vi "gCode_analyseReceivedMessage.vi"(10 "UI_Data":T2={"controlTabState"=[], "pathToSTLFiles"=path "", "availableObjs"=[], "objectNames"=[], "addedObjs"=[], "selectedObj"={"Name"="", "objectFiles"=[], "center"={"X"=0.0, "Y"=0.0, "Z"=0.0}, "extent"={"X"=0.0, "Y"=0.0, "Z"=0.0}, "allowedMotion"=enum."XY", "mountOn"=enum."yArm", "Movements"=[], "extraInfo"=[], "hasPOI?"=FALSE, "POI"={"X"=0.0, "Y"=0.0, "Z"=0.0}, "posOffset"={"X"=0.0, "Y"=0.0, "Z"=0.0}, "referenceNum"=refnum}, "3DPictureObjRef"=refnum, "yPOI_0"={"X"=0.0, "Y"=0.0, "Z"=0.0}, "yPOI"={"X"=0.0, "Y"=0.0, "Z"=0.0}, "yPOI_Added?"=FALSE, "breadBoard_00"={"X"=0.0, "Y"=0.0, "Z"=0.0}, "breadBoardOriginOffset"={"X"=0.0, "Y"=0.0, "Z"=0.0}, "XYtranslateObjControls"=[], "ZtranslateObjControls"=[], "pBot_controls"=[], "pBot_VISA"="", "commandLog"="", "pBotConnected?"=FALSE, "pBot_currentEEPROMsettings"="", "realTimeInfoControls"=[], "pBot_tempSensor1"=0.0, "pBot_tempSensor2"=0.0, "realTimeInfoTextColor"=[], "disconnectPBot_Event"=refnum, "needToHomeY?"=FALSE, "pBot_relativePositioning"=FALSE, "pBot_minPos"={"X"=0.0, "Y"=0.0, "Z"=0.0}, "pBot_maxPos"={"X"=0.0, "Y"=0.0, "Z"=0.0}, "pBot_homeOffset"={"X"=0.0, "Y"=0.0, "Z"=0.0}, "textColorGreen"=9174826, "textColorRed"=16750216, "textColorGray"=9868950, "transVisualizationControls"=[], "needToHomeXY?"=FALSE, "pBot_minScanRegion"={"X"=0.0, "Y"=0.0, "Z"=0.0}, "pBot_maxScanRegion"={"X"=0.0, "Y"=0.0, "Z"=0.0}, "pBot_scanN"={"X"=0, "Y"=0, "Z"=0}, "connectedInstruments"=[], "isScanning?"=FALSE, "Wavelengths"=[], "usb2000p_controlRefs"=[], "3DPictureRef"=refnum}, 11 "pBotMessageData":T1={"commandID"=" ", "gCode"=" ", "extraInfo"=" ", "originatingCommandID"=" ", "error"={"status"=FALSE, "code"=0, "source"=""}}) -> (0 "error Out":errorcluster, 2 "UI_Data Out":T2={"controlTabState"=[], "pathToSTLFiles"=path "", "availableObjs"=[], "objectNames"=[], "addedObjs"=[], "selectedObj"={"Name"="", "objectFiles"=[], "center"={"X"=0.0, "Y"=0.0, "Z"=0.0}, "extent"={"X"=0.0, "Y"=0.0, "Z"=0.0}, "allowedMotion"=enum."XY", "mountOn"=enum."yArm", "Movements"=[], "extraInfo"=[], "hasPOI?"=FALSE, "POI"={"X"=0.0, "Y"=0.0, "Z"=0.0}, "posOffset"={"X"=0.0, "Y"=0.0, "Z"=0.0}, "referenceNum"=refnum}, "3DPictureObjRef"=refnum, "yPOI_0"={"X"=0.0, "Y"=0.0, "Z"=0.0}, "yPOI"={"X"=0.0, "Y"=0.0, "Z"=0.0}, "yPOI_Added?"=FALSE, "breadBoard_00"={"X"=0.0, "Y"=0.0, "Z"=0.0}, "breadBoardOriginOffset"={"X"=25.4, "Y"=12.7, "Z"=12.7}, "XYtranslateObjControls"=[], "ZtranslateObjControls"=[], "pBot_controls"=[], "pBot_VISA"="", "commandLog"="", "pBotConnected?"=FALSE, "pBot_currentEEPROMsettings"="", "realTimeInfoControls"=[], "pBot_tempSensor1"=0.0, "pBot_tempSensor2"=0.0, "realTimeInfoTextColor"=[], "disconnectPBot_Event"=refnum, "needToHomeY?"=FALSE, "pBot_relativePositioning"=FALSE, "pBot_minPos"={"X"=0.0, "Y"=0.0, "Z"=0.0}, "pBot_maxPos"={"X"=0.0, "Y"=0.0, "Z"=0.0}, "pBot_homeOffset"={"X"=0.0, "Y"=0.0, "Z"=0.0}, "textColorGreen"=9174826, "textColorRed"=16750216, "textColorGray"=9868950, "transVisualizationControls"=[], "needToHomeXY?"=FALSE, "pBot_minScanRegion"={"X"=0.0, "Y"=0.0, "Z"=0.0}, "pBot_maxScanRegion"={"X"=0.0, "Y"=0.0, "Z"=0.0}, "pBot_scanN"={"X"=0, "Y"=0, "Z"=0}, "connectedInstruments"=[], "isScanning?"=FALSE, "Wavelengths"=[], "usb2000p_controlRefs"=[], "3DPictureRef"=refnum}, 3 "messageOut":string)   [LabVIEW 2015]
uses:
  controls/UI Data.ctl
  processedObjectInfo.ctl
  controls/scanInstrumentInfo.ctl
  controls/pBotMessageData.ctl
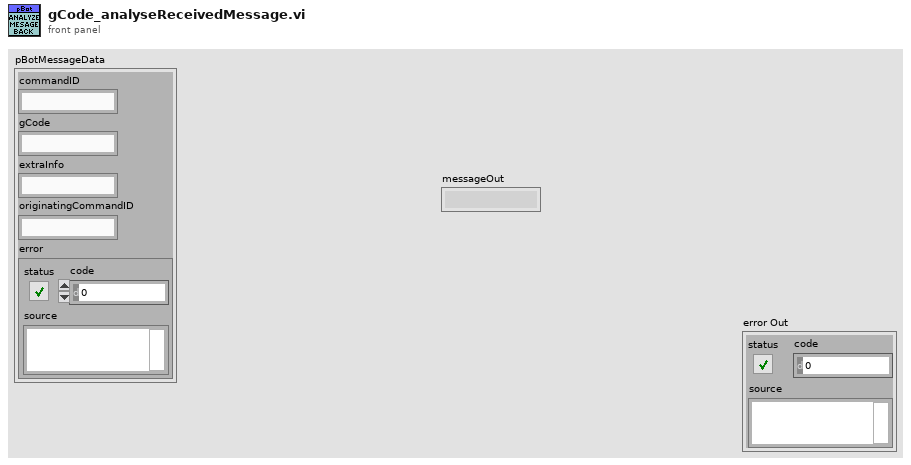
[diagram p1: front panel]
types:
  T1 = typedef "pBotMessageData.ctl" = cluster{"commandID":string, "gCode":string, "extraInfo":string, "originatingCommandID":string, "error":errorcluster}
  T2 = typedef "UI Data.ctl" = cluster{"controlTabState":bool[], "pathToSTLFiles":path, "availableObjs":T3[], "objectNames":string[], "addedObjs":T3[], "selectedObj":T3, "3DPictureObjRef":refnum<vi>, "yPOI_0":cluster{"X":dbl, "Y":dbl, "Z":dbl}, "yPOI":cluster{"X":dbl, "Y":dbl, "Z":dbl}, "yPOI_Added?":bool, "breadBoard_00":cluster{"X":dbl, "Y":dbl, "Z":dbl}, "breadBoardOriginOffset":cluster{"X":dbl, "Y":dbl, "Z":dbl}, "XYtranslateObjControls":refnum<vi>[], "ZtranslateObjControls":refnum<vi>[], "pBot_controls":refnum<vi>[], "pBot_VISA":refnum<visa-resource-name>, "commandLog":string, "pBotConnected?":bool, "pBot_currentEEPROMsettings":string, "realTimeInfoControls":refnum<vi>[], "pBot_tempSensor1":dbl, "pBot_tempSensor2":dbl, "realTimeInfoTextColor":u32[], "disconnectPBot_Event":refnum<user-event>, "needToHomeY?":bool, "pBot_relativePositioning":bool, "pBot_minPos":cluster{"X":dbl, "Y":dbl, "Z":dbl}, "pBot_maxPos":cluster{"X":dbl, "Y":dbl, "Z":dbl}, "pBot_homeOffset":cluster{"X":dbl, "Y":dbl, "Z":dbl}, "textColorGreen":u32, "textColorRed":u32, "textColorGray":u32, "transVisualizationControls":refnum<vi>[], "needToHomeXY?":bool, "pBot_minScanRegion":cluster{"X":sgl, "Y":sgl, "Z":sgl}, "pBot_maxScanRegion":cluster{"X":sgl, "Y":sgl, "Z":sgl}, "pBot_scanN":cluster{"X":u16, "Y":u16, "Z":u16}, "connectedInstruments":T4[], "isScanning?":bool, "Wavelengths":dbl[], "usb2000p_controlRefs":refnum<vi>[], "3DPictureRef":refnum<vi>}
  T3 = typedef "processedObjectInfo.ctl" = cluster{"Name":string, "objectFiles":cluster{"Location":path, "Color":cluster{"R":dbl, "G":dbl, "B":dbl, "A":dbl}}[], "center":cluster{"X":dbl, "Y":dbl, "Z":dbl}, "extent":cluster{"X":dbl, "Y":dbl, "Z":dbl}, "allowedMotion":enum16{"XY", "Z"}, "mountOn":enum16{"yArm", "breadBoard"}, "Movements":cluster{"Type":enum16{"rr", "ra", "tr", "ta"}, "vector":cluster{"X":dbl, "Y":dbl, "Z":dbl}, "scalar":dbl}[], "extraInfo":cluster{"parameter":string, "dataType":string, "vector":cluster{"X":dbl, "Y":dbl, "Z":dbl}, "scalar":dbl}[], "hasPOI?":bool, "POI":cluster{"X":dbl, "Y":dbl, "Z":dbl}, "posOffset":cluster{"X":dbl, "Y":dbl, "Z":dbl}, "referenceNum":refnum<vi>}
  T4 = typedef "scanInstrumentInfo.ctl" = cluster{"Name":string, "VISAname":refnum<visa-resource-name>, "1D_dataArraySize":u16, "extraInfo":variant, "error":errorcluster}
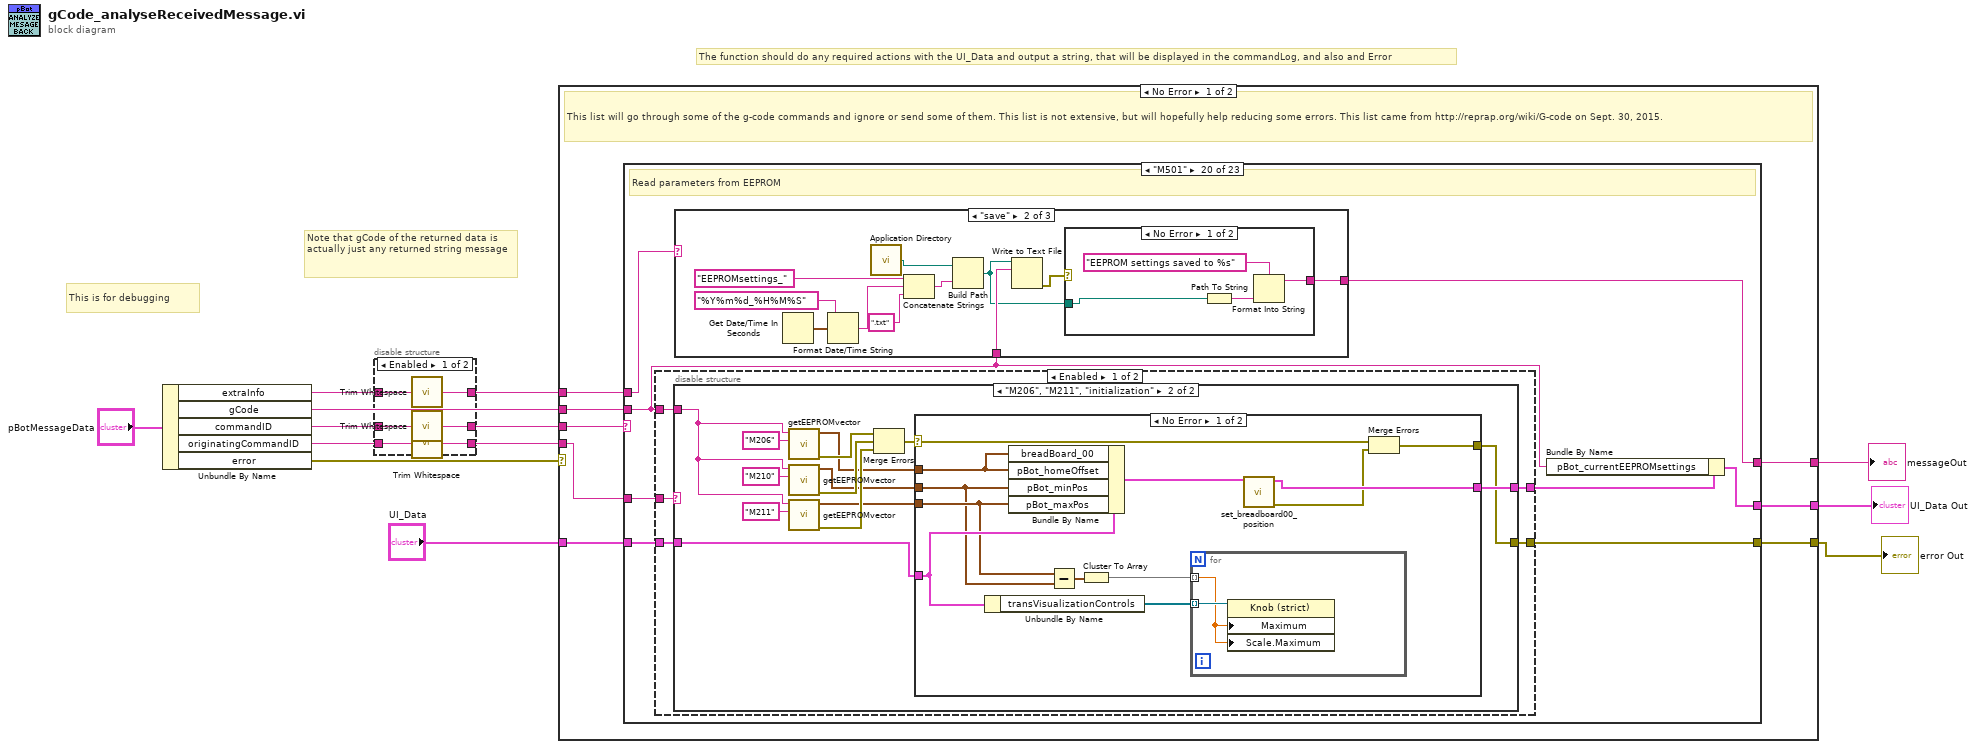
[diagram p0: block diagram]
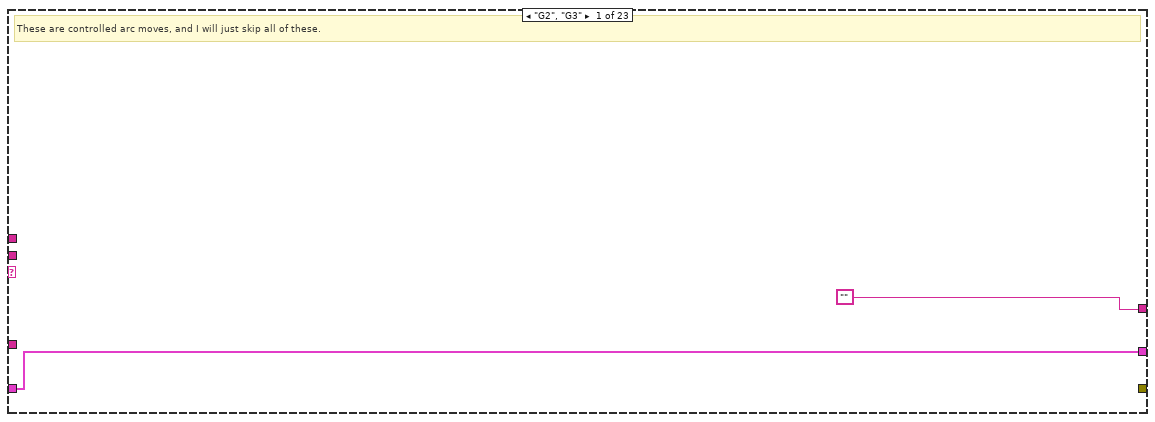
[diagram p3: hidden frame]
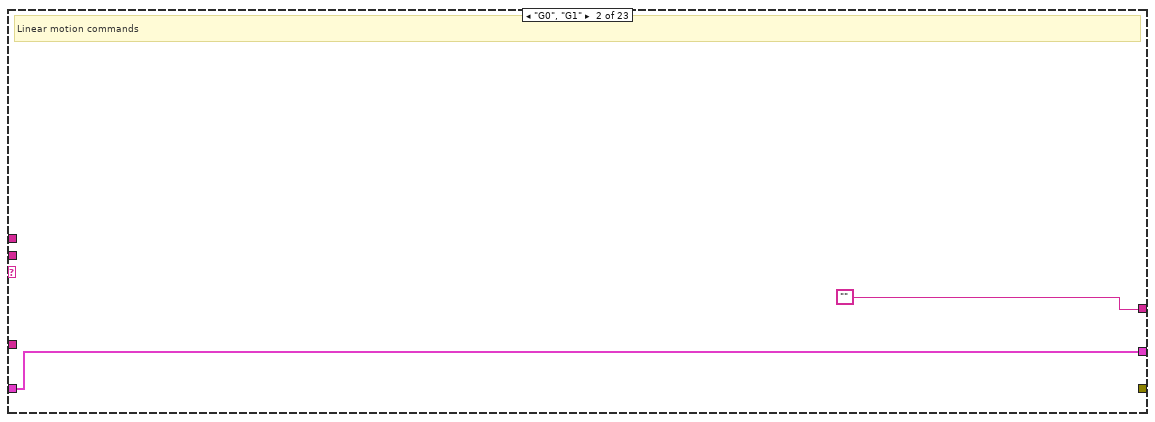
[diagram p4: hidden frame]
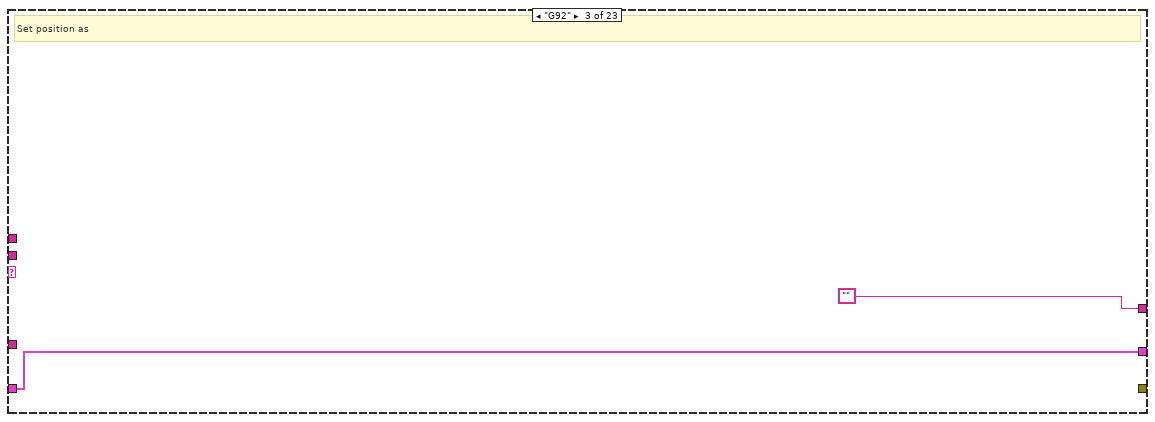
[diagram p5: hidden frame]
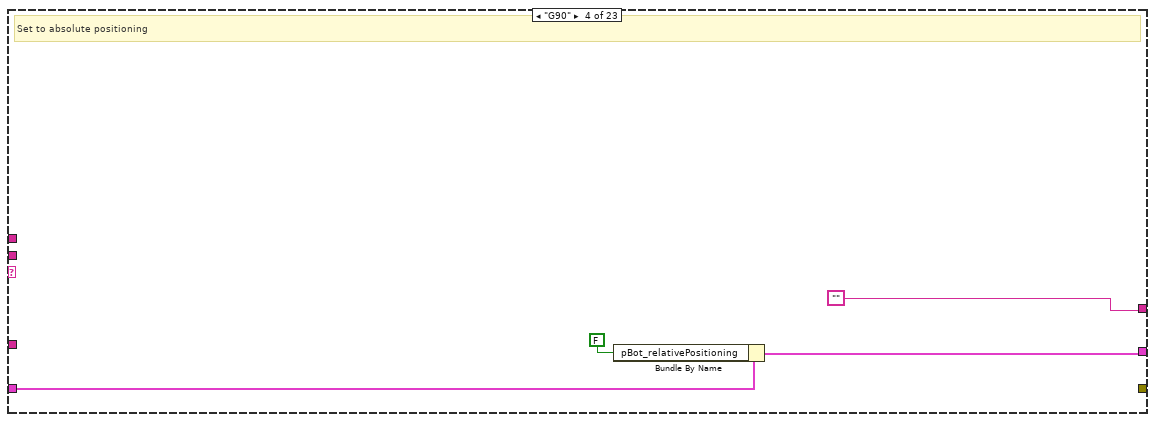
[diagram p6: hidden frame]
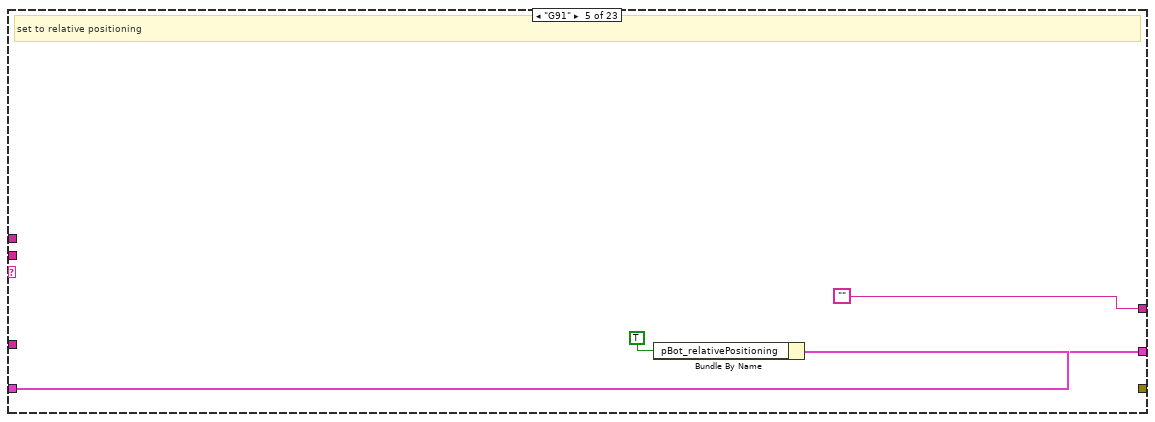
[diagram p7: hidden frame]
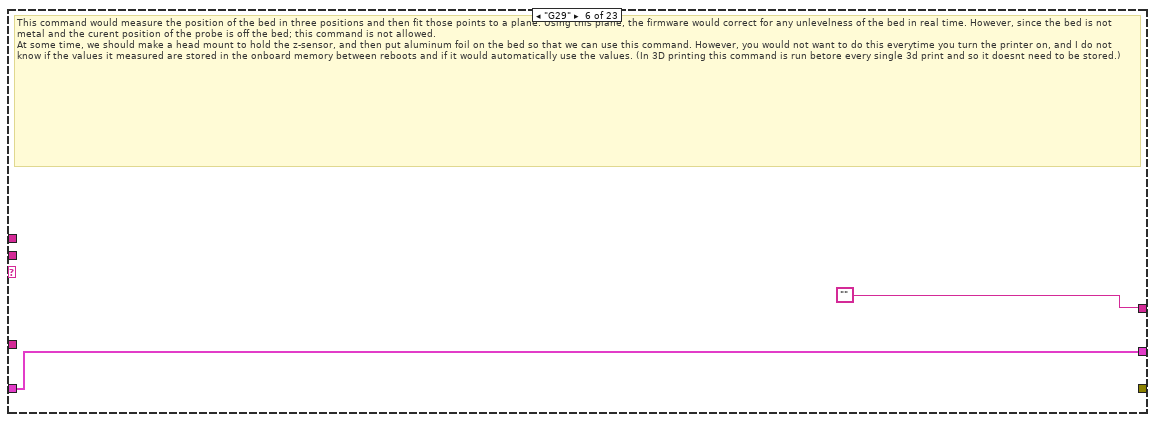
[diagram p8: hidden frame]
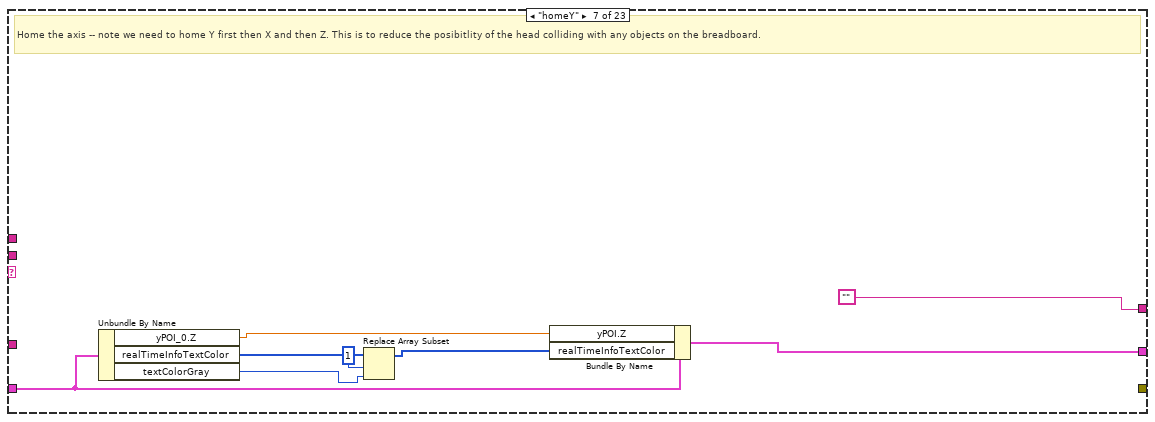
[diagram p9: hidden frame]
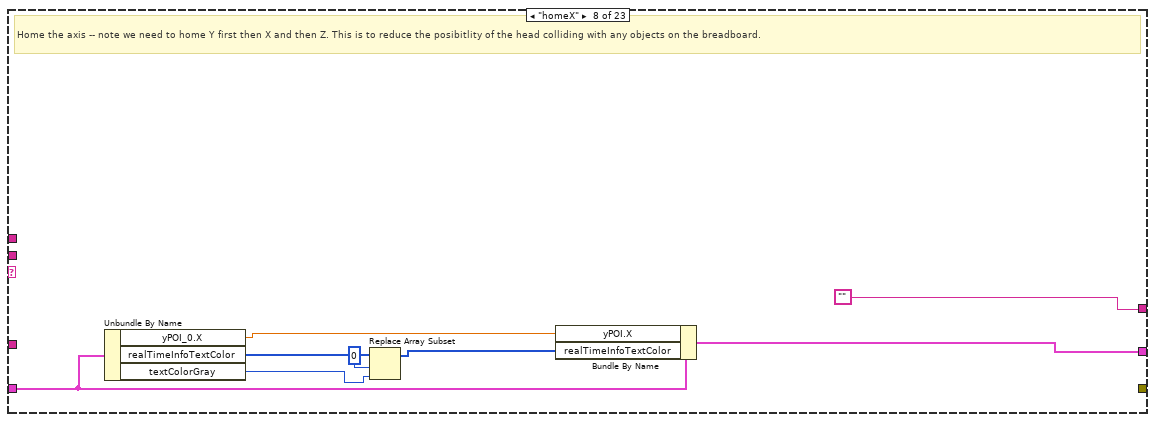
[diagram p10: hidden frame]
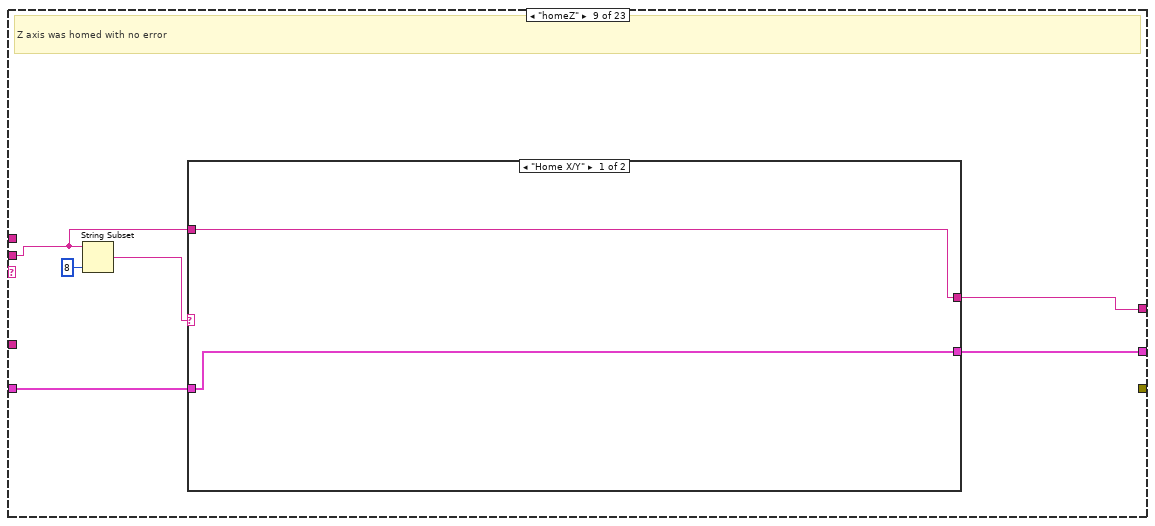
[diagram p11: hidden frame]
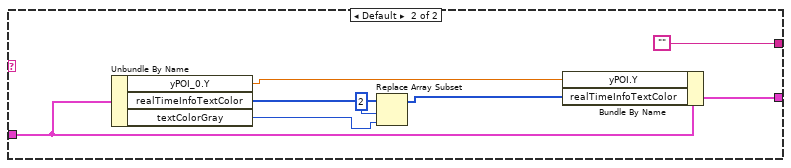
[diagram p12: hidden frame]
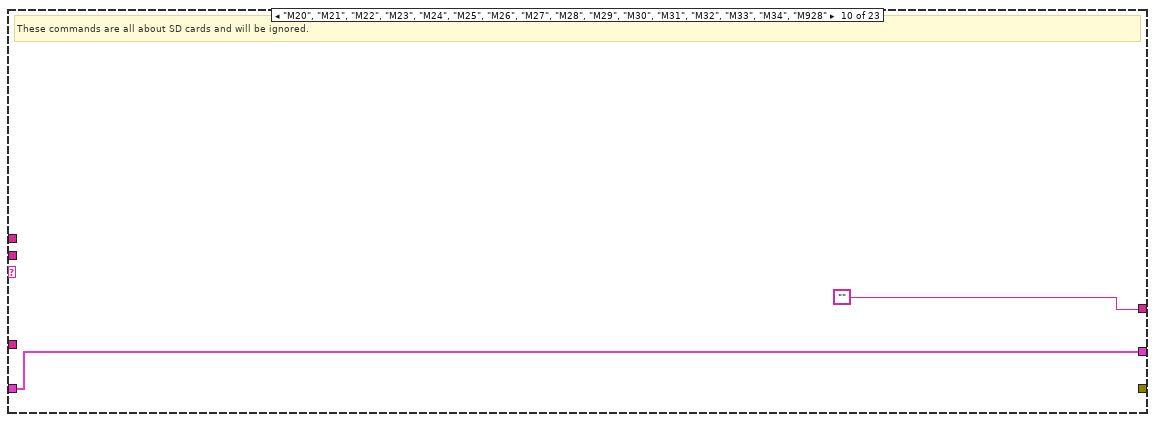
[diagram p13: hidden frame]
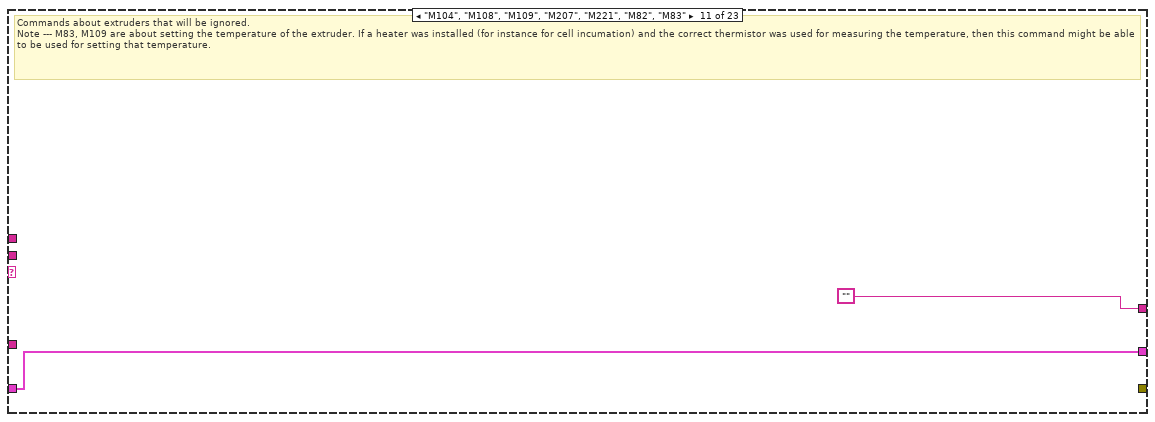
[diagram p14: hidden frame]
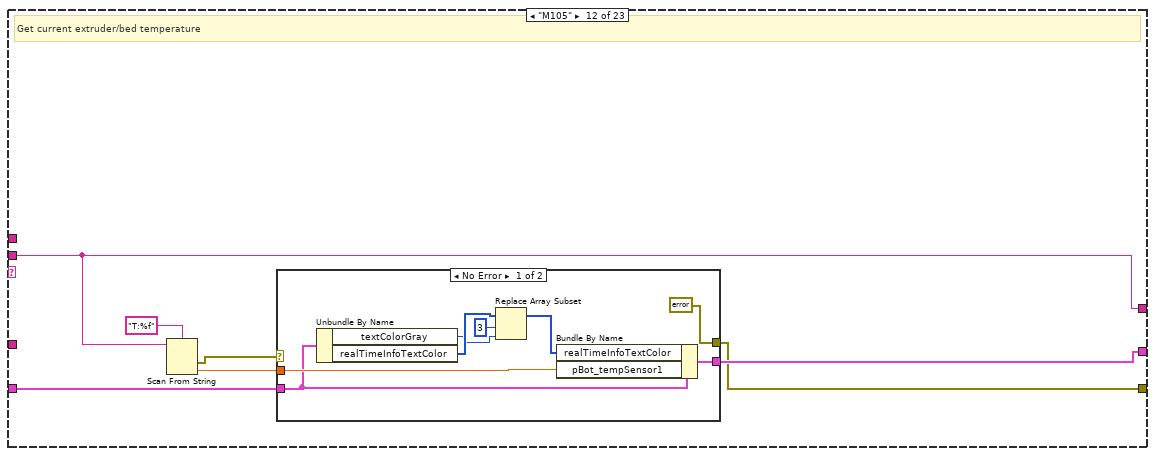
[diagram p15: hidden frame]
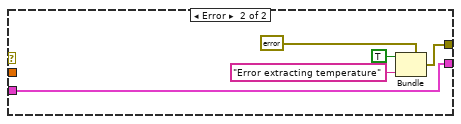
[diagram p16: hidden frame]
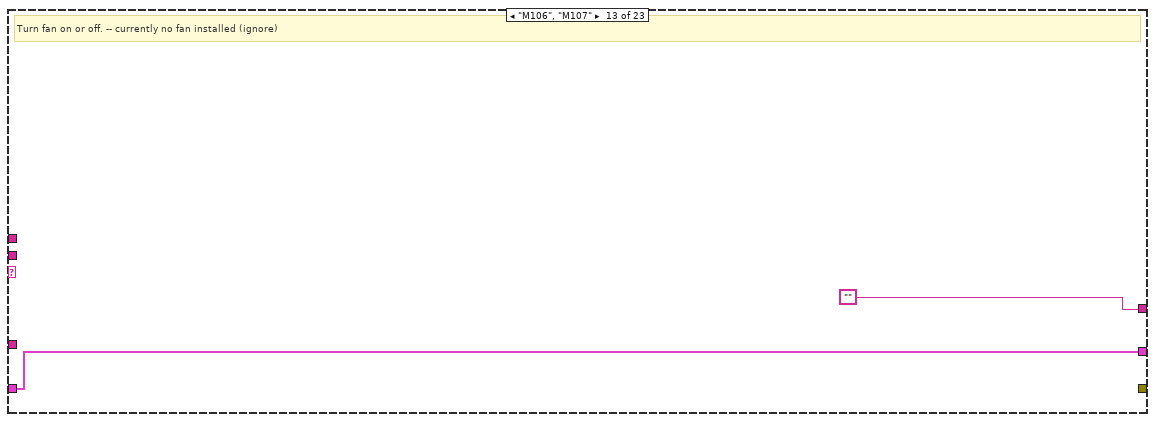
[diagram p17: hidden frame]
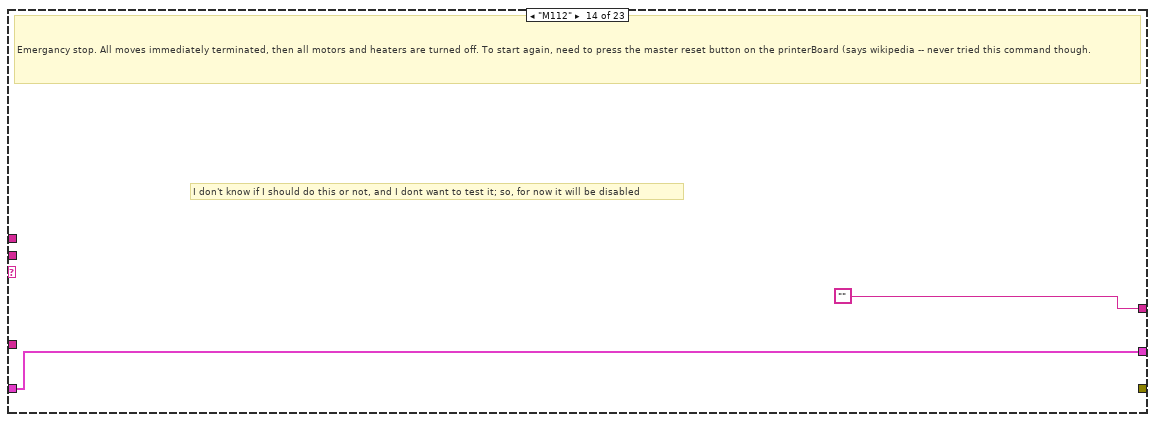
[diagram p18: hidden frame]
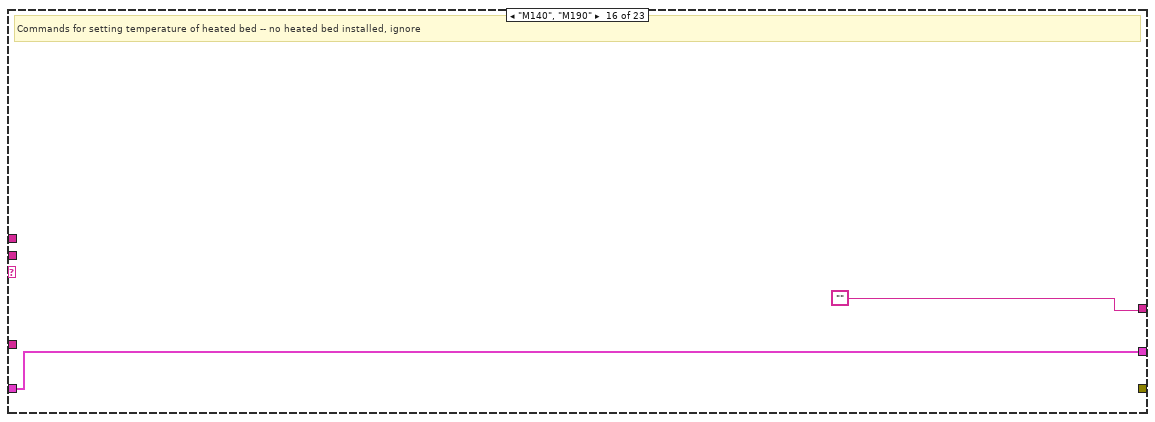
[diagram p20: hidden frame]
diagram:
  # "This is for debugging"
  # "Note that gCode of the returned data is actually just any returned string message"
  # "The function should do any required actions with the UI_Data and output a string, that will be displayed in the commandLog, and also and Error"
  n1 = Unbundle By Name("pBotMessageData") -> ("extraInfo"=w2:string, "gCode"=w11:string, "commandID"=w3:string, "originatingCommandID"=w6:string, "error"=w13:errorcluster)
  n2 = disable-structure shown="Enabled" {
    disable-tunnel: w6 -> [w19 w20]
    disable-tunnel: [w18 w20] -> w5
    disable-tunnel: [w17 w21] -> w4
    disable-tunnel: w3 -> [w16 w21]
    disable-tunnel: w2 -> [w15 w22]
    disable-tunnel: [w14 w22] -> w1
    frame Enabled {
      n3 = call <vilib>:"Trim Whitespace.vi"("string"=w15) -> ("trimmed string"=w14:string)  [unwired: 1 in]
      n4 = call <vilib>:"Trim Whitespace.vi"("string"=w16) -> ("trimmed string"=w17:string)  [unwired: 1 in]
      n5 = call <vilib>:"Trim Whitespace.vi"("string"=w19) -> ("trimmed string"=w18:string)  [unwired: 1 in]
    }
    frame Disabled {
    }
  }
  n6 = case shown="No Error" w13 {
    selector: w13 -> [_ w188]
    tunnel: [w28 w191] -> w10
    tunnel: w4 -> [w30 w193]
    tunnel: "UI_Data" -> [w29 w192]
    tunnel: w11 -> [w27 w190]
    tunnel: [w26 w189] -> w8
    tunnel: [w25 w187] -> w9
    tunnel: w1 -> [w24 _]
    tunnel: w5 -> [w23 _]
    frame No Error {
      # "This list will go through some of the g-code commands and ignore or send some of them. This list is not extensive, but will hopefully help reducing some errors. This list came from http://reprap.org/wiki/G-code on Sept. 30, 2015."
      n7 = case shown="\"M501\"" w30 {
        tunnel: w29 -> [w32 w34 w36 w40 w43 w46 w50 w57 w68 w80 w81 w87 w104 w106 w107 w110 w111 w114 w115 w124 w182 w184 w186]
        tunnel: [w32 w34 w36 w39 w42 w46 w49 w58 w67 w80 w81 w85 w104 w106 w107 w110 w111 w114 w115 w122 w182 w184 w186] -> w25
        tunnel: ["" "" "" "" "" "" "" "" w66 "" "" w83 "" "" w108 "" "" "" w116 w121 w181 "" w185] -> w28
        tunnel: w27 -> [_ _ _ _ _ _ _ _ w63 _ _ w83 _ _ w108 _ _ _ w116 w119 w181 _ w185]
        tunnel: [_ _ _ _ _ _ _ _ _ _ _ w84 _ _ _ _ _ _ _ w120 _ _ _] -> w26
        tunnel: w24 -> [_ _ _ _ _ _ _ _ _ _ _ _ _ _ _ _ _ _ _ w118 _ _ _]
        tunnel: w23 -> [_ _ _ _ _ _ _ _ _ _ _ _ _ _ _ _ _ _ _ w117 _ _ _]
        frame "G2", "G3" {
          # "These are controlled arc moves, and I will just skip all of these."
        }
        frame "G0", "G1" {
          # "Linear motion commands"
        }
        frame "G92" {
          # "Set position as"
        }
        frame "G90" {
          # "Set to absolute positioning"
          n8 = Bundle By Name(cluster=w40, "pBot_relativePositioning"=FALSE) -> (w39:T2)
        }
        frame "G91" {
          # "set to relative positioning"
          n9 = Bundle By Name(cluster=w43, "pBot_relativePositioning"=TRUE) -> (w42:T2)
        }
        frame "G29" {
          # "This command would measure the position of the bed in three positions and then fit those points to a plane. Using this plane, the firmware would correct for any unlevelness of the bed in real time. However, since the bed is not metal and the curent position of the probe is off the bed; this command is not allowed.\nAt some time, we should make a head mount to hold the z-sensor, and then put aluminum foil on the bed so that we can use this command. However, you would not want to do this everytime you turn the printer on, and I do not know if the values it measured are stored in the onboard memory between reboots and if it would automatically use the values. (In 3D printing this command is run betore every single 3d print and so it doesnt need to be stored.)"
        }
        frame "homeY" {
          # "Home the axis -- note we need to home Y first then X and then Z. This is to reduce the posibitlity of the head colliding with any objects on the breadboard."
          n10 = Unbundle By Name(w50) -> ("yPOI_0.Z"=w47:dbl, "realTimeInfoTextColor"=w54:u32[], "textColorGray"=w52:u32)
          n11 = Replace Array Subset(array=w54, new element=w52, index=1) -> (w51:u32[])
          n12 = Bundle By Name(cluster=w50, "yPOI.Z"=w47, "realTimeInfoTextColor"=w51) -> (w49:T2)
        }
        frame "homeX" {
          # "Home the axis -- note we need to home Y first then X and then Z. This is to reduce the posibitlity of the head colliding with any objects on the breadboard."
          n13 = Unbundle By Name(w57) -> ("yPOI_0.X"=w55:dbl, "realTimeInfoTextColor"=w62:u32[], "textColorGray"=w60:u32)
          n14 = Replace Array Subset(array=w62, new element=w60, index=0) -> (w59:u32[])
          n15 = Bundle By Name(cluster=w57, "yPOI.X"=w55, "realTimeInfoTextColor"=w59) -> (w58:T2)
        }
        frame "homeZ" {
          # "Z axis was homed with no error"
          n16 = String Subset(string=w63, length (rest)=8 ("length (rest)")) -> (substring=w64:string)  [unwired: 1 in]
          n17 = case shown="\"Home X/Y\"" w64 {
            tunnel: w68 -> [w70 w78]
            tunnel: [w70 w73] -> w67
            tunnel: [w69 ""] -> w66
            tunnel: w63 -> [w69 _]
            frame "Home X/Y" {
            }
            frame Default {
              n18 = Unbundle By Name(w78) -> ("yPOI_0.Y"=w71:dbl, "realTimeInfoTextColor"=w77:u32[], "textColorGray"=w75:u32)
              n19 = Replace Array Subset(array=w77, new element=w75, index=2) -> (w74:u32[])
              n20 = Bundle By Name(cluster=w78, "yPOI.Y"=w71, "realTimeInfoTextColor"=w74) -> (w73:T2)
            }
          }
        }
        frame "M20", "M21", "M22", "M23", "M24", "M25", "M26", "M27", "M28", "M29", "M30", "M31", "M32", "M33", "M34", "M928" {
          # "These commands are all about SD cards and will be ignored."
        }
        frame "M104", "M108", "M109", "M207", "M221", "M82", "M83" {
          # "Commands about extruders that will be ignored.\nNote --- M83, M109 are about setting the temperature of the extruder. If a heater was installed (for instance for cell incumation) and the correct thermistor was used for measuring the temperature, then this command might be able to be used for setting that temperature."
        }
        frame "M105" {
          # "Get current extruder/bed temperature"
          n21 = Scan From String(format string="T:%f", input string=w83) -> (error out=w88:errorcluster, output 1=w86:dbl)  [unwired: 3 in, 2 out]
          n22 = case shown="No Error" w88 {
            tunnel: w87 -> [w94 w102]
            tunnel: [w97 w102] -> w85
            tunnel: w86 -> [w96 _]
            tunnel: [errorcluster {"status"=FALSE, "code"=0, "source"=""} ("error constant") w98] -> w84
            frame No Error {
              n23 = Unbundle By Name(w94) -> ("textColorGray"=w91:u32, "realTimeInfoTextColor"=w92:u32[])
              n24 = Replace Array Subset(array=w92, new element=w91, index=3) -> (w90:u32[])
              n25 = Bundle By Name(cluster=w94, "realTimeInfoTextColor"=w90, "pBot_tempSensor1"=w96) -> (w97:T2)
            }
            frame Error {
              n26 = Bundle(cluster=errorcluster {"status"=FALSE, "code"=0, "source"=""} ("error constant"), "status"=TRUE, "source"="Error extracting temperature") -> (w98:errorcluster)  [unwired: 1 in]
            }
          }
        }
        frame "M106", "M107" {
          # "Turn fan on or off. -- currently no fan installed (ignore)"
        }
        frame "M112" {
          # "I don't know if I should do this or not, and I dont want to test it; so, for now it will be disabled"
          # "Emergancy stop. All moves immediately terminated, then all motors and heaters are turned off. To start again, need to press the master reset button on the printerBoard (says wikipedia -- never tried this command though."
        }
        frame "M114" {
          # "Get current position."
        }
        frame "M140", "M190" {
          # "Commands for setting temperature of heated bed -- no heated bed installed, ignore"
        }
        frame "M206" {
          # "If this value was changed than that means that the homePos_Offset has changed and we need to update yPOI_Home and yPOI_Current. This update will be done in the M501 case, since M501 is sent after every M206."
        }
        frame "M210", "M211" {
        }
        frame "M502" {
          # "Resets all tunable parameters to factory reset values."
        }
        frame "M501" {
          # "Read parameters from EEPROM"
          n27 = disable-structure shown="Enabled" {
            disable-tunnel: w124 -> [w129 w162]
            disable-tunnel: [w128 w162] -> w123
            disable-tunnel: [w127 _] -> w120
            disable-tunnel: w119 -> [w126 _]
            disable-tunnel: w117 -> [w125 _]
            frame Enabled {
              n28 = case shown="\"M206\", \"M211\", \"initialization\"" w125 {
                tunnel: w129 -> [w130 w135]
                tunnel: [w130 w134] -> w128
                tunnel: [errorcluster {"status"=FALSE, "code"=0, "source"=""} ("error IO") w133] -> w127
                tunnel: w126 -> [_ w132]
                frame Default {
                }
                frame "M206", "M211", "initialization" {
                  n29 = call "getEEPROMvector.vi"("vectorName"="M206", "EEPROM_Settings"=w132) -> ("error out"=w142:errorcluster, "vectorOut"=w138:cluster{dbl, dbl, dbl})  [unwired: 8 in]
                  n30 = call "getEEPROMvector.vi"("vectorName"="M210", "EEPROM_Settings"=w132) -> ("error out"=w141:errorcluster, "vectorOut"=w137:cluster{dbl, dbl, dbl})  [unwired: 8 in]
                  n31 = call "getEEPROMvector.vi"("vectorName"="M211", "EEPROM_Settings"=w132) -> ("error out"=w140:errorcluster, "vectorOut"=w136:cluster{dbl, dbl, dbl})  [unwired: 8 in]
                  n32 = Merge Errors(w142, w141, w140) -> (w139:errorcluster)
                  n33 = case shown="No Error" w139 {
                    selector: w139 -> [w147 w160]
                    tunnel: w138 -> [w151 _]
                    tunnel: w137 -> [w155 _]
                    tunnel: w136 -> [w156 _]
                    tunnel: w135 -> [w157 w161]
                    tunnel: [w149 w161] -> w134
                    tunnel: [w146 w160] -> w133
                    frame No Error {
                      n34 = Unbundle By Name(w157) -> ("transVisualizationControls"=w154:refnum<vi>[])
                      n35 = Bundle By Name(cluster=w157, "breadBoard_00"=w151, "pBot_homeOffset"=w151, "pBot_minPos"=w155, "pBot_maxPos"=w156) -> (w150:T2)
                      n36 = Subtract(x=w156, y=w155) -> (x-y=w153:cluster{dbl, dbl, dbl})
                      n37 = Cluster To Array(cluster=w153) -> (array=w152:dbl[])
                      n38 = for {
                        tunnel: w154 -> [w159] mode=indexing
                        tunnel: w152 -> [w158] mode=indexing
                        n39 = property class="Knob (strict)"(reference=w159, "Maximum"=w158, "Scale.Maximum"=w158) -> ()  [unwired: 1 in, 2 out]
                      }
                      n40 = call "set_breadboard00_position.vi"("UI_Data"=w150) -> ("error out"=w148:errorcluster, "UI_Data out"=w149:T2)  [unwired: 9 in]
                      n41 = Merge Errors(w147, w148) -> (w146:errorcluster)
                    }
                    frame Error {
                    }
                  }
                }
              }
            }
            frame Disabled {
            }
          }
          n42 = case shown="\"save\"" w118 {
            tunnel: w119 -> [w163 w167 _]
            tunnel: [w163 w164 ""] -> w121
            frame Default {
            }
            frame "save" {
              n43 = Get Date/Time In Seconds() -> (seconds since 1Jan1904=w173:timestamp)
              n44 = Format Date/Time String(time format string (%c)="%Y%m%d_%H%M%S", seconds (now)=w173) -> (date/time string=w171:string)  [unwired: 1 in]
              n45 = call <vilib>:"Application Directory.vi"() -> ("Application Directory"=w168:path)
              n46 = Concatenate Strings("EEPROMsettings_" ("name or relative path"), w171, ".txt" ("string")) -> (w169:string)
              n47 = Build Path(base path=w168, name or relative path=w169) -> (appended path=w165:path)
              n48 = Write to Text File(file (use dialog)=w165, text=w167) -> (error out=w166:errorcluster)  [unwired: 2 in, 2 out]
              n49 = case shown="No Error" w166 {
                tunnel: w165 -> [w176 _]
                tunnel: [w175 "Warning! EEPROM settings not sucessfully saved!" ("name or relative path")] -> w164
                frame No Error {
                  n50 = Path To String(path=w176) -> (string=w177:string)
                  n51 = Format Into String(format string="EEPROM settings saved to %s" ("name or relative path"), w177) -> (resulting string=w175:string)  [unwired: 2 in, 1 out]
                }
                frame Error {
                }
              }
            }
            frame "noDisplay" {
            }
          }
          n52 = Bundle By Name(cluster=w123, "pBot_currentEEPROMsettings"=w119) -> (w122:T2)
        }
        frame "M500" {
          # "Save parameters to EEPROM"
        }
        frame "M600", "M605", "M665", "M668", "M999" {
          # "other commands to ignore"
        }
        frame Default {
          # "An unknown command was send, just pass along the message (gCode)"
        }
      }
    }
    frame Error {
      (unwired) ""
      # "An error occured (other than a Timeout) while getting a responce from the plasmaBot\nThis list will go through some of the g-code commands and ignore or send some of them. This list is not extensive, but will hopefully help reducing some errors. This list came from http://reprap.org/wiki/G-code on Sept. 30, 2015."
      n53 = case shown="\"M20\", \"M21\", \"M22\", \"M23\", \"M24\", \"M25\", \"M26\", \"M27\", \"M28\", \"M29\", \"M30\", \"M31\", \"M32\", \"M33\", \"M34\", \"M928\"" w193 {
        tunnel: w192 -> [w195 w198 w209 w214 w218 w221 w226 w234 w248 w251 w253 w257 w265 w268 w271 w274 w277 w278 w283 w286 w289]
        tunnel: [w195 w197 w209 w213 w217 w221 w225 w235 w243 w251 w253 w256 w265 w268 w271 w274 w277 w278 w283 w286 w289] -> w187
        tunnel: ["" "" "" "" "" "" "" "" "" "" "" "" "" "" "" "" "" "" "" "" ""] -> w191
        tunnel: w190 -> [_ _ _ _ _ _ _ _ _ _ _ _ _ _ _ _ _ _ _ _ _]
        tunnel: [_ errorcluster {"status"=TRUE, "code"=0, "source"="Error! An error occured while moving. The system may be in an undermined state. Please proceed with caution."} ("error constant") _ errorcluster {"status"=TRUE, "code"=0, "source"="Error! An error occured while trying to change to absolute positioning. The sytem may be in an undetermined state. Proceed with great caution!"} ("error constant") errorcluster {"status"=TRUE, "code"=0, "source"="Error! An error occured while trying to change to relative positioning. The sytem may be in an undetermined state. Proceed with great caution!"} ("error constant") _ errorcluster {"status"=TRUE, "code"=0, "source"="Error! An error occured while homing the Y axis. The system may be in an undermined state. Please proceed with caution."} ("error constant") errorcluster {"status"=TRUE, "code"=0, "source"="Error! An error occured while homing the X axis. The system may be in an undermined state. Please proceed with caution."} ("error constant") errorcluster {"status"=TRUE, "code"=0, "source"="Error! An error occured while homing the Z axis. The system may be in an undermined state. Please proceed with caution."} ("error constant") w249 w252 errorcluster {"status"=TRUE, "code"=0, "source"="An error occured while getting the current temperatures."} ("error constant") w263 w266 w270 w272 w275 w279 w281 w284 w288] -> w189
        tunnel: w188 -> [_ _ _ _ _ _ _ _ _ w249 w252 _ w263 w266 w270 w272 w275 w279 w281 w284 w288]
        frame "G2", "G3" {
          # "These are controlled arc moves, and I will just skip all of these."
        }
        frame "G0", "G1" {
          # "Linear motion commands"
          n54 = Unbundle By Name(w198) -> ("realTimeInfoTextColor"=w206:u32[], "textColorRed"=w200:u32)
          n55 = Replace Array Subset(array=w206, new element=w200, index=0) -> (w204:u32[])
          n56 = Replace Array Subset(array=w204, new element=w200, index=1) -> (w202:u32[])
          n57 = Replace Array Subset(array=w202, new element=w200, index=2) -> (w199:u32[])
          n58 = Bundle By Name(cluster=w198, "realTimeInfoTextColor"=w199) -> (w197:T2)
        }
        frame "G92" {
          # "Set position as"
        }
        frame "G90" {
          # "Set to absolute positioning"
          n59 = Bundle By Name(cluster=w214, "pBot_relativePositioning"=FALSE) -> (w213:T2)
        }
        frame "G91" {
          # "set to relative positioning"
          n60 = Bundle By Name(cluster=w218, "pBot_relativePositioning"=TRUE) -> (w217:T2)
        }
        frame "G29" {
          # "This command would measure the position of the bed in three positions and then fit those points to a plane. Using this plane, the firmware would correct for any unlevelness of the bed in real time. However, since the bed is not metal and the curent position of the probe is off the bed; this command is not allowed.\nAt some time, we should make a head mount to hold the z-sensor, and then put aluminum foil on the bed so that we can use this command. However, you would not want to do this everytime you turn the printer on, and I do not know if the values it measured are stored in the onboard memory between reboots and if it would automatically use the values. (In 3D printing this command is run betore every single 3d print and so it doesnt need to be stored.)"
        }
        frame "homeY" {
          # "Home the axis -- note we need to home Y first then X and then Z. This is to reduce the posibitlity of the head colliding with any objects on the breadboard."
          n61 = Unbundle By Name(w226) -> ("yPOI_0.Z"=w223:dbl, "realTimeInfoTextColor"=w230:u32[], "textColorRed"=w228:u32)
          n62 = Replace Array Subset(array=w230, new element=w228, index=1) -> (w227:u32[])
          n63 = Bundle By Name(cluster=w226, "yPOI.Z"=w223, "realTimeInfoTextColor"=w227) -> (w225:T2)
        }
        frame "homeX" {
          # "Home the axis -- note we need to home Y first then X and then Z. This is to reduce the posibitlity of the head colliding with any objects on the breadboard."
          n64 = Unbundle By Name(w234) -> ("yPOI_0.X"=w232:dbl, "realTimeInfoTextColor"=w239:u32[], "textColorRed"=w237:u32)
          n65 = Replace Array Subset(array=w239, new element=w237, index=0) -> (w236:u32[])
          n66 = Bundle By Name(cluster=w234, "yPOI.X"=w232, "realTimeInfoTextColor"=w236) -> (w235:T2)
        }
        frame "homeZ" {
          # "Z axis was homed with no error"
          n67 = Unbundle By Name(w248) -> ("yPOI_0.Y"=w241:dbl, "realTimeInfoTextColor"=w247:u32[], "textColorRed"=w245:u32)
          n68 = Replace Array Subset(array=w247, new element=w245, index=2) -> (w244:u32[])
          n69 = Bundle By Name(cluster=w248, "yPOI.Y"=w241, "realTimeInfoTextColor"=w244) -> (w243:T2)
        }
        frame "M20", "M21", "M22", "M23", "M24", "M25", "M26", "M27", "M28", "M29", "M30", "M31", "M32", "M33", "M34", "M928" {
          # "These commands are all about SD cards and will be ignored."
        }
        frame "M104", "M108", "M109", "M207", "M221", "M82", "M83" {
          # "Commands about extruders that will be ignored.\nNote --- M83, M109 are about setting the temperature of the extruder. If a heater was installed (for instance for cell incumation) and the correct thermistor was used for measuring the temperature, then this command might be able to be used for setting that temperature."
        }
        frame "M105" {
          # "Get current extruder/bed temperature"
          n70 = Unbundle By Name(w257) -> ("textColorRed"=w259:u32, "realTimeInfoTextColor"=w260:u32[])
          n71 = Replace Array Subset(array=w260, new element=w259, index=3) -> (w258:u32[])
          n72 = Bundle By Name(cluster=w257, "realTimeInfoTextColor"=w258) -> (w256:T2)
        }
        frame "M106", "M107" {
          # "Turn fan on or off. -- currently no fan installed (ignore)"
        }
        frame "M112" {
          # "I don't know if I should do this or not, and I dont want to test it; so, for now it will be disabled"
          # "Emergancy stop. All moves immediately terminated, then all motors and heaters are turned off. To start again, need to press the master reset button on the printerBoard (says wikipedia -- never tried this command though."
        }
        frame "M114" {
          # "Get current position."
        }
        frame "M140", "M190" {
          # "Commands for setting temperature of heated bed -- no heated bed installed, ignore"
        }
        frame "M502" {
          # "Resets all tunable parameters to factory reset values."
        }
        frame "M501" {
          # "Read parameters from EEPROM"
        }
        frame "M500" {
          # "Save parameters to EEPROM"
        }
        frame "M600", "M605", "M665", "M668", "M999" {
          # "other commands to ignore"
        }
        frame Default {
          # "IF the command is not in this case structure, then ask the user to make sure they want to send the command to the printerboard"
        }
      }
    }
  }
  "messageOut" <- w10
  "UI_Data Out" <- w9
  "error Out" <- w8
